vi "LondonMetData.vi"(5 "Met Data File Path":path=path "C:/Users/Hesham/Documents/GitHub/LabVIEW/Wind Analysis/LondonCombined.csv") -> (0 "k":dbl[][](array[numeric]), 1 "c":dbl[][](array[numeric]), 2 "p":dbl[][](array[numeric]))   [LabVIEW 2018]
uses:
  <vilib>/Utility/file.llb/Read Delimited Spreadsheet (DBL).vi
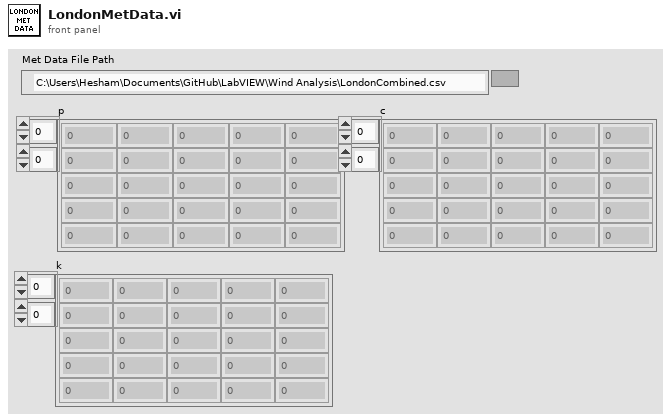
[diagram p1: front panel]
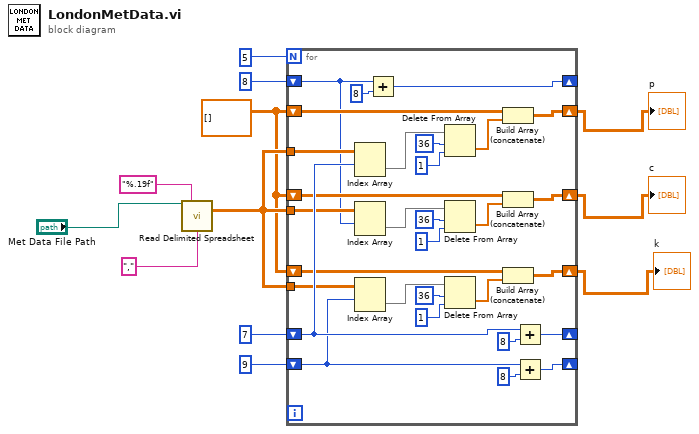
[diagram p0: block diagram]
diagram:
  w6 = dbl[][] []
  n1 = call-poly <vilib>:"Read Delimited Spreadsheet.vi"("file path (dialog if empty)"="Met Data File Path", "format (%.3f)"="%.19f", "delimiter (\\t)"="," ("delimiter (\\t)")) -> ("all rows"=w7:dbl[][])  [unwired: 7 in, 5 out]
  n2 = for {
    N: 5 -> [_]
    tunnel: w7 -> [w39]
    shift-right: [w36] -> w5
    shift-left: w6 -> [w35]
    shift-right: [w34] -> _
    shift-left: 7 -> [w33]
    shift-right: [w26] -> w4
    shift-left: w6 -> [w27]
    tunnel: w7 -> [w25]
    shift-right: [w23] -> _
    shift-left: 8 -> [w24]
    shift-right: [w19] -> w3
    shift-left: w6 -> [w18]
    tunnel: w7 -> [w20]
    shift-right: [w22] -> _
    shift-left: 9 -> [w21]
    n3 = Index Array(array=w39, index (row)=w33) -> (element=w42:dbl[])  [unwired: 1 in]
    n4 = Index Array(array=w25, index (row)=w24) -> (element=w28:dbl[])  [unwired: 1 in]
    n5 = Index Array(array=w20, index (row)=w21) -> (element=w17:dbl[])  [unwired: 1 in]
    n6 = Add(x=w24, y=8) -> (x+y=w23:i32)
    n7 = Delete From Array(array=w42, length=36, index=1 ("length")) -> (deleted portion=w37:dbl[])  [unwired: 1 out]
    n8 = Delete From Array(array=w28, length=36, index=1 ("length")) -> (deleted portion=w32:dbl[])  [unwired: 1 out]
    n9 = Delete From Array(array=w17, length=36, index=1 ("length")) -> (deleted portion=w13:dbl[])  [unwired: 1 out]
    n10 = Build Array (concatenate)(w35, w37) -> (w36:dbl[][])
    n11 = Build Array (concatenate)(w27, w32) -> (w26:dbl[][])
    n12 = Build Array (concatenate)(w18, w13) -> (w19:dbl[][])
    n13 = Add(x=w33, y=8) -> (x+y=w34:i32)
    n14 = Add(x=w21, y=8) -> (x+y=w22:i32)
  }
  "p" <- w5
  "c" <- w4
  "k" <- w3
